vi "Create All Message Queues.vi"(8 "error in (no error)":errorcluster) -> (0 "error out":errorcluster, 3 "Message Queues out":T1)   [LabVIEW 2017, in "Message Queue.lvlib"]
doc: "This VI creates and initializes all the message queues for your application. If your application requires more than one message queue, right-click the \"Message Queues\" constant above and select Open Type Def. Add the new Message Queue(s) to the type definition, then initialize them in this VI."
uses:
  Message Queue.lvlib
  All Message Queues.ctl
  Message Cluster.ctl
  Enqueue Message (Single).vi
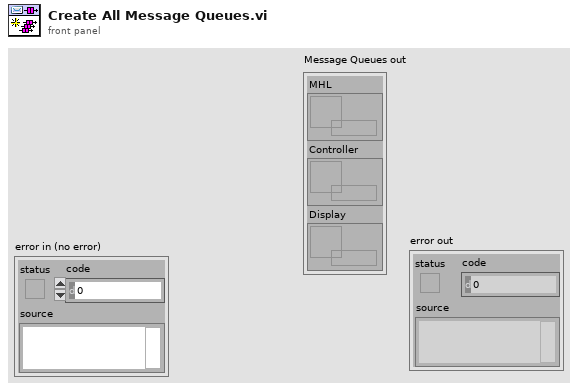
[diagram p1: front panel]
types:
  T1 = typedef "Message Queue.lvlib/All Message Queues.ctl" = cluster{"MHL":refnum<queue>, "Controller":refnum<queue>, "Display":refnum<queue>}
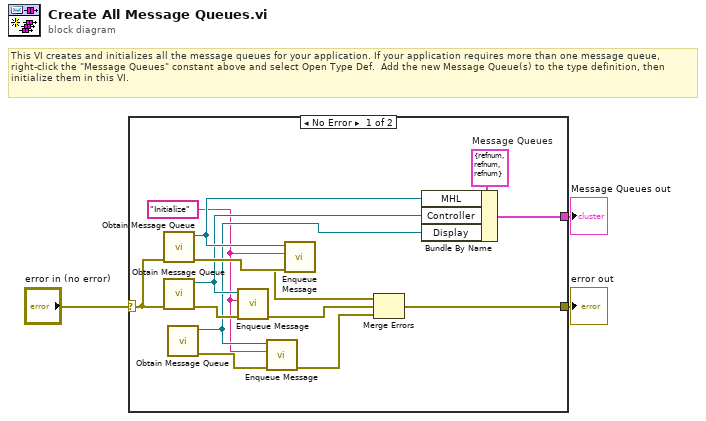
[diagram p0: block diagram]
diagram:
  # "This VI creates and initializes all the message queues for your application. If your application requires more than one message queue, right-click the \"Message Queues\" constant above and select Open Type Def.  Add the new Message Queue(s) to the type definition, then initialize them in this VI."
  n1 = case shown="No Error" "error in (no error)" {
    selector: "error in (no error)" -> [w12 w18]
    tunnel: [w4 w18] -> w3
    tunnel: [w16 _] -> w2
    frame No Error {
      w6 = "Initialize" ("Message")
      w17 = T1 {"MHL"=refnum, "Controller"=refnum, "Display"=refnum}  # Message Queues
      n2 = call "Obtain Message Queue.vi"("error in (no error)"=w12) -> ("error out"=w15:errorcluster, "Message Queue"=w14:refnum<queue>)  [unwired: 9 in]
      n3 = call "Obtain Message Queue.vi"("error in (no error)"=w12) -> ("error out"=w13:errorcluster, "Message Queue"=w9:refnum<queue>)  [unwired: 9 in]
      n4 = call "Obtain Message Queue.vi"() -> ("error out"=w8:errorcluster, "Message Queue"=w7:refnum<queue>)  [unwired: 10 in]
      n5 = call-poly "Enqueue Message.vi"("error in (no error)"=w13, "Message"=w6, "Message Queue"=w9) -> ("error out"=w10:errorcluster)  [unwired: 7 in, 1 out]
      n6 = call-poly "Enqueue Message.vi"("error in (no error)"=w8, "Message"=w6, "Message Queue"=w7) -> ("error out"=w5:errorcluster)  [unwired: 7 in, 1 out]
      n7 = call-poly "Enqueue Message.vi"("error in (no error)"=w15, "Message"=w6, "Message Queue"=w14) -> ("error out"=w11:errorcluster)  [unwired: 7 in, 1 out]
      n8 = Merge Errors(w11, w10, w5) -> (w4:errorcluster)
      n9 = Bundle By Name(cluster=w17, "MHL"=w14, "Controller"=w9, "Display"=w7) -> (w16:T1)
    }
    frame Error {
    }
  }
  "Message Queues out" <- w2
  "error out" <- w3
